vi "Play.vi"(8 "error in (no error)":errorcluster, 9 "fileName":string, 10 "audioType":string, 11 "AudioPlayer in":refnum<class "AudioPlayer.lvclass">) -> (0 "error out":errorcluster, 3 "AudioPlayer out":refnum<class "AudioPlayer.lvclass">)   [LabVIEW 2018, in "AudioPlayer.lvclass"]
uses:
  AudioPlayer.lvclass
  AudioPlayer.lvclass/AudioPlayer.ctl
  ConsoleOut/Print Options.ctl
  Media Adapter/MediaAdapter.lvclass
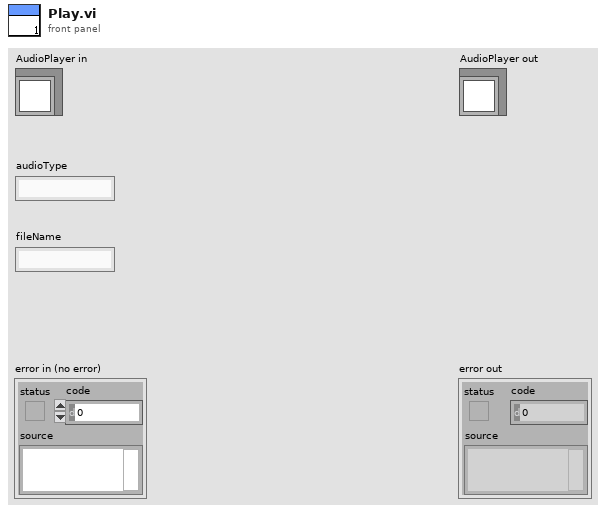
[diagram p1: front panel]
types:
  T1 = typedef "Print Options.ctl" = enum16{"Create", "Get Reference", "Print", "Print Header", "Close"}
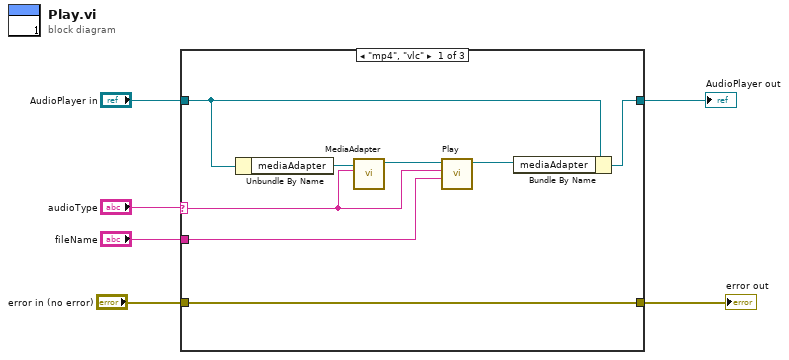
[diagram p0: block diagram]
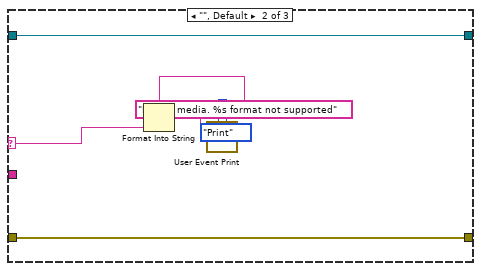
[diagram p2: hidden frame]
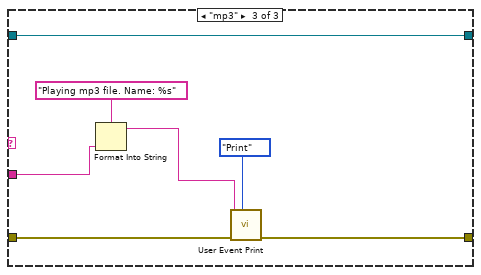
[diagram p3: hidden frame]
diagram:
  n1 = case shown="\"mp4\", \"vlc\"" "audioType" {
    selector: "audioType" -> [w8 w18 _]
    tunnel: [w12 w20 w27] -> w6
    tunnel: "AudioPlayer in" -> [w14 w20 w27]
    tunnel: "fileName" -> [w9 _ w25]
    tunnel: "error in (no error)" -> [w7 w15 w22]
    tunnel: [w7 w15 w21] -> w1
    frame "mp4", "vlc" {
      n2 = Unbundle By Name(w14) -> ("mediaAdapter"=w13:refnum<class "MediaAdapter.lvclass">)
      n3 = call "MediaAdapter.vi"("audioType"=w8, "MediaAdapter in"=w13) -> ("MediaAdapter out"=w11:refnum<class "MediaAdapter.lvclass">)  [unwired: 8 in, 1 out]
      n4 = call-dynamic "Play.vi"("fileName"=w9, "audioType"=w8, "MediaAdapter in"=w11) -> ("MediaAdapter out"=w10:refnum<class "MediaAdapter.lvclass">)  [unwired: 7 in, 1 out]
      n5 = Bundle By Name(cluster=w14, "mediaAdapter"=w10) -> (w12:refnum<class "AudioPlayer.lvclass">)
    }
    frame "", Default {
      n6 = Format Into String(format string="Invalid media. %s format not supported", w18) -> (resulting string=w17:string)  [unwired: 2 in, 1 out]
      n7 = call "User Event Print.vi"("Options"=Print_Options."Print", "String to Print"=w17) -> ()  [unwired: 8 in, 2 out]
    }
    frame "mp3" {
      n8 = Format Into String(format string="Playing mp3 file. Name: %s", w25) -> (resulting string=w24:string)  [unwired: 2 in, 1 out]
      n9 = call "User Event Print.vi"("Options"=Print_Options."Print", "error in (no error)"=w22, "String to Print"=w24) -> ("error out"=w21:errorcluster)  [unwired: 7 in, 1 out]
    }
  }
  "error out" <- w1
  "AudioPlayer out" <- w6
